vi "Calculate Microphone Sensitivity.vi"(9 "microphone sensitivity (dBFS)":dbl, 10 "measured sound level (dBSPL)":dbl, 11 "reference sound level (dBSPL)":dbl) -> (3 "calculated microphone sensitivity (dBFS)":dbl)   [LabVIEW 2022 SP3]
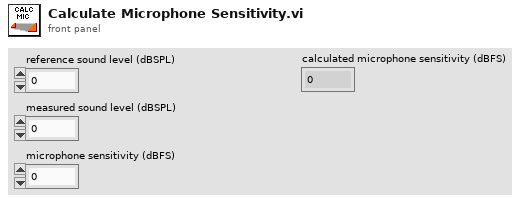
[diagram p1: front panel]
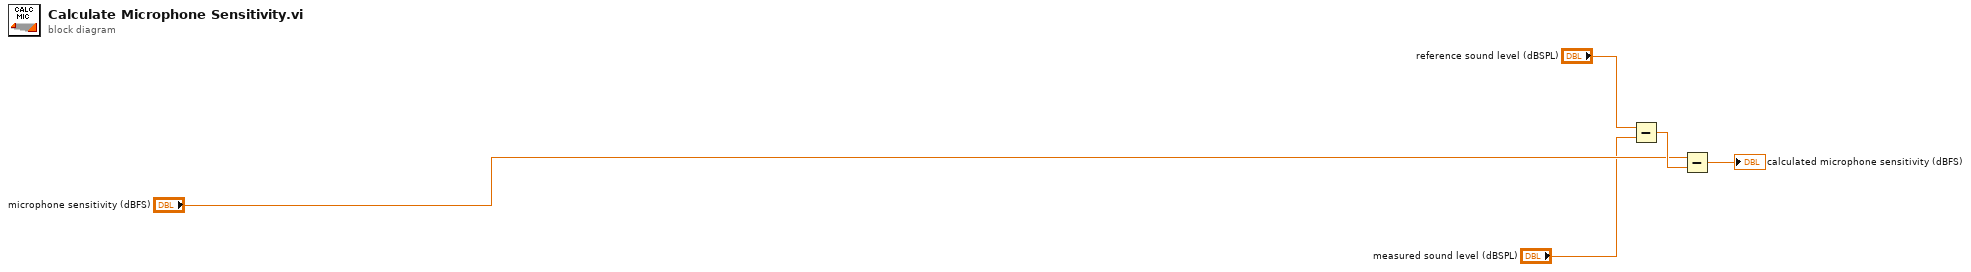
[diagram p0: block diagram]
diagram:
  n1 = Subtract(x="reference sound level (dBSPL)", y="measured sound level (dBSPL)") -> (x-y=w4:dbl)
  n2 = Subtract(x="microphone sensitivity (dBFS)", y=w4) -> (x-y=→"calculated microphone sensitivity (dBFS)":dbl)
